vi "FMA1600A Meter Standard Accuracy.vi"(8 "Error In":errorcluster, 11 "Meter Accuracy Option 1":T1) -> (0 "Error Out":errorcluster, 2 "Full Scale Accuracy %":string, 3 "Reading Accuracy %":string)   [LabVIEW 2018]
uses:
  Type Definitions/FMA1600A Meter Accuracy Options.ctl
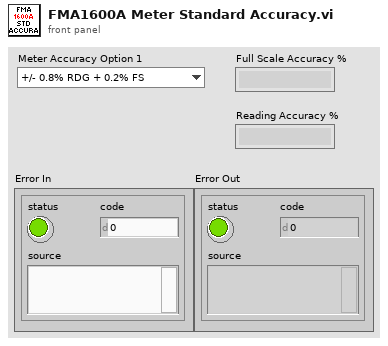
[diagram p1: front panel]
types:
  T1 = typedef "FMA1600A Meter Accuracy Options.ctl" = enum16{"+/- 0.8% RDG + 0.2% FS", "+/- 0.4% RDG + 0.2% FS"}
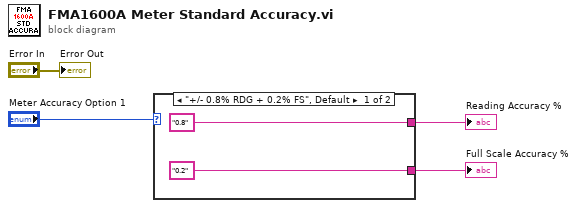
[diagram p0: block diagram]
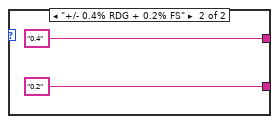
[diagram p2: hidden frame]
diagram:
  n1 = case shown="\"+/- 0.8% RDG + 0.2% FS\", Default" "Meter Accuracy Option 1" {
    tunnel: ["0.8" "0.4"] -> w4
    tunnel: ["0.2" "0.2"] -> w3
    frame "+/- 0.8% RDG + 0.2% FS", Default {
    }
    frame "+/- 0.4% RDG + 0.2% FS" {
    }
  }
  "Reading Accuracy %" <- w4
  "Full Scale Accuracy %" <- w3
  "Error Out" <- "Error In"
